vi "ziExample-Module-Sweeper.vi"() -> ()   [LabVIEW 2009]
doc: "Control a Zurich instrument device via the LabOne Labview API. \nRequirements: Zurich Instruments MFLI, HF2 or UHFLI \nThis example shows how to start a sweeper module and retrieve data.\n\n© Zurich Instruments AG, www.zhinst.com"
uses:
  <instrlib>/Zurich Instruments LabOne/Public/Modules/ziTypeModSweeperImpedanceWave.ctl
  <instrlib>/Zurich Instruments LabOne/Public/Modules/ziTypeModSweeperDemodWave.ctl
  <instrlib>/Zurich Instruments LabOne/Public/Modules/ziTypeModSweeperDoubleWave.ctl
  <instrlib>/Zurich Instruments LabOne/Public/Modules/ziModSetValueDouble.vi
  <instrlib>/Zurich Instruments LabOne/Public/Modules/ziModSetValueBinary.vi
  <instrlib>/Zurich Instruments LabOne/Public/Modules/ziModSetValueDoubleArray.vi
  <instrlib>/Zurich Instruments LabOne/Public/Configure/ziSetValueDoubleArray.vi
  <instrlib>/Zurich Instruments LabOne/Public/Modules/ziModGetDoubleData.vi
  <instrlib>/Zurich Instruments LabOne/Public/Modules/ziModGetSweeperData.vi
  <instrlib>/Zurich Instruments LabOne/Zurich Instruments LabOne.lvlib
panel:
  out "SweeperDoubleWaveArray":T1[](array[typedef]) {"bandwidthMode" format="%f"; "flags" format="%f"; "sampleFormat" format="%f"; "sweepMode" format="%f"; "sampleCount" format="%f"; "timestamp" format="%f"}
  out "SweeperDemodWaveArray":T2[](array[typedef]) {"bandwidthMode" format="%f"; "flags" format="%f"; "sampleFormat" format="%f"; "sweepMode" format="%f"; "sampleCount" format="%f"; "timestamp" format="%f"}
  out "SweeperImpedanceWaveArray":T3[](array[typedef]) {"bandwidthMode" format="%f"; "flags" format="%f"; "sampleFormat" format="%f"; "sweepMode" format="%f"; "sampleCount" format="%f"; "timestamp" format="%f"}
  out "Error Out":errorcluster
  in  "Address":string="DEV"
  out "Settings":T4
  out "Selected Device":string
  in  "subscribepath":string="demods/0/sample" caption="Subscribe Path"
  out "Sweeper Phase":cluster{"grid":dbl[], "r_avg":dbl[]}(graph)
  out "Sweeper R":cluster{"grid":dbl[], "r_avg":dbl[]}(graph)
  # "ziExample-SweepModul.vi\nRequirements: HF2LI, UHFLI or MFLI\nsee block diagram for VI description"
  # "Tested Devices:\n- HF2LI\n- UHFLI\n- MFLI"
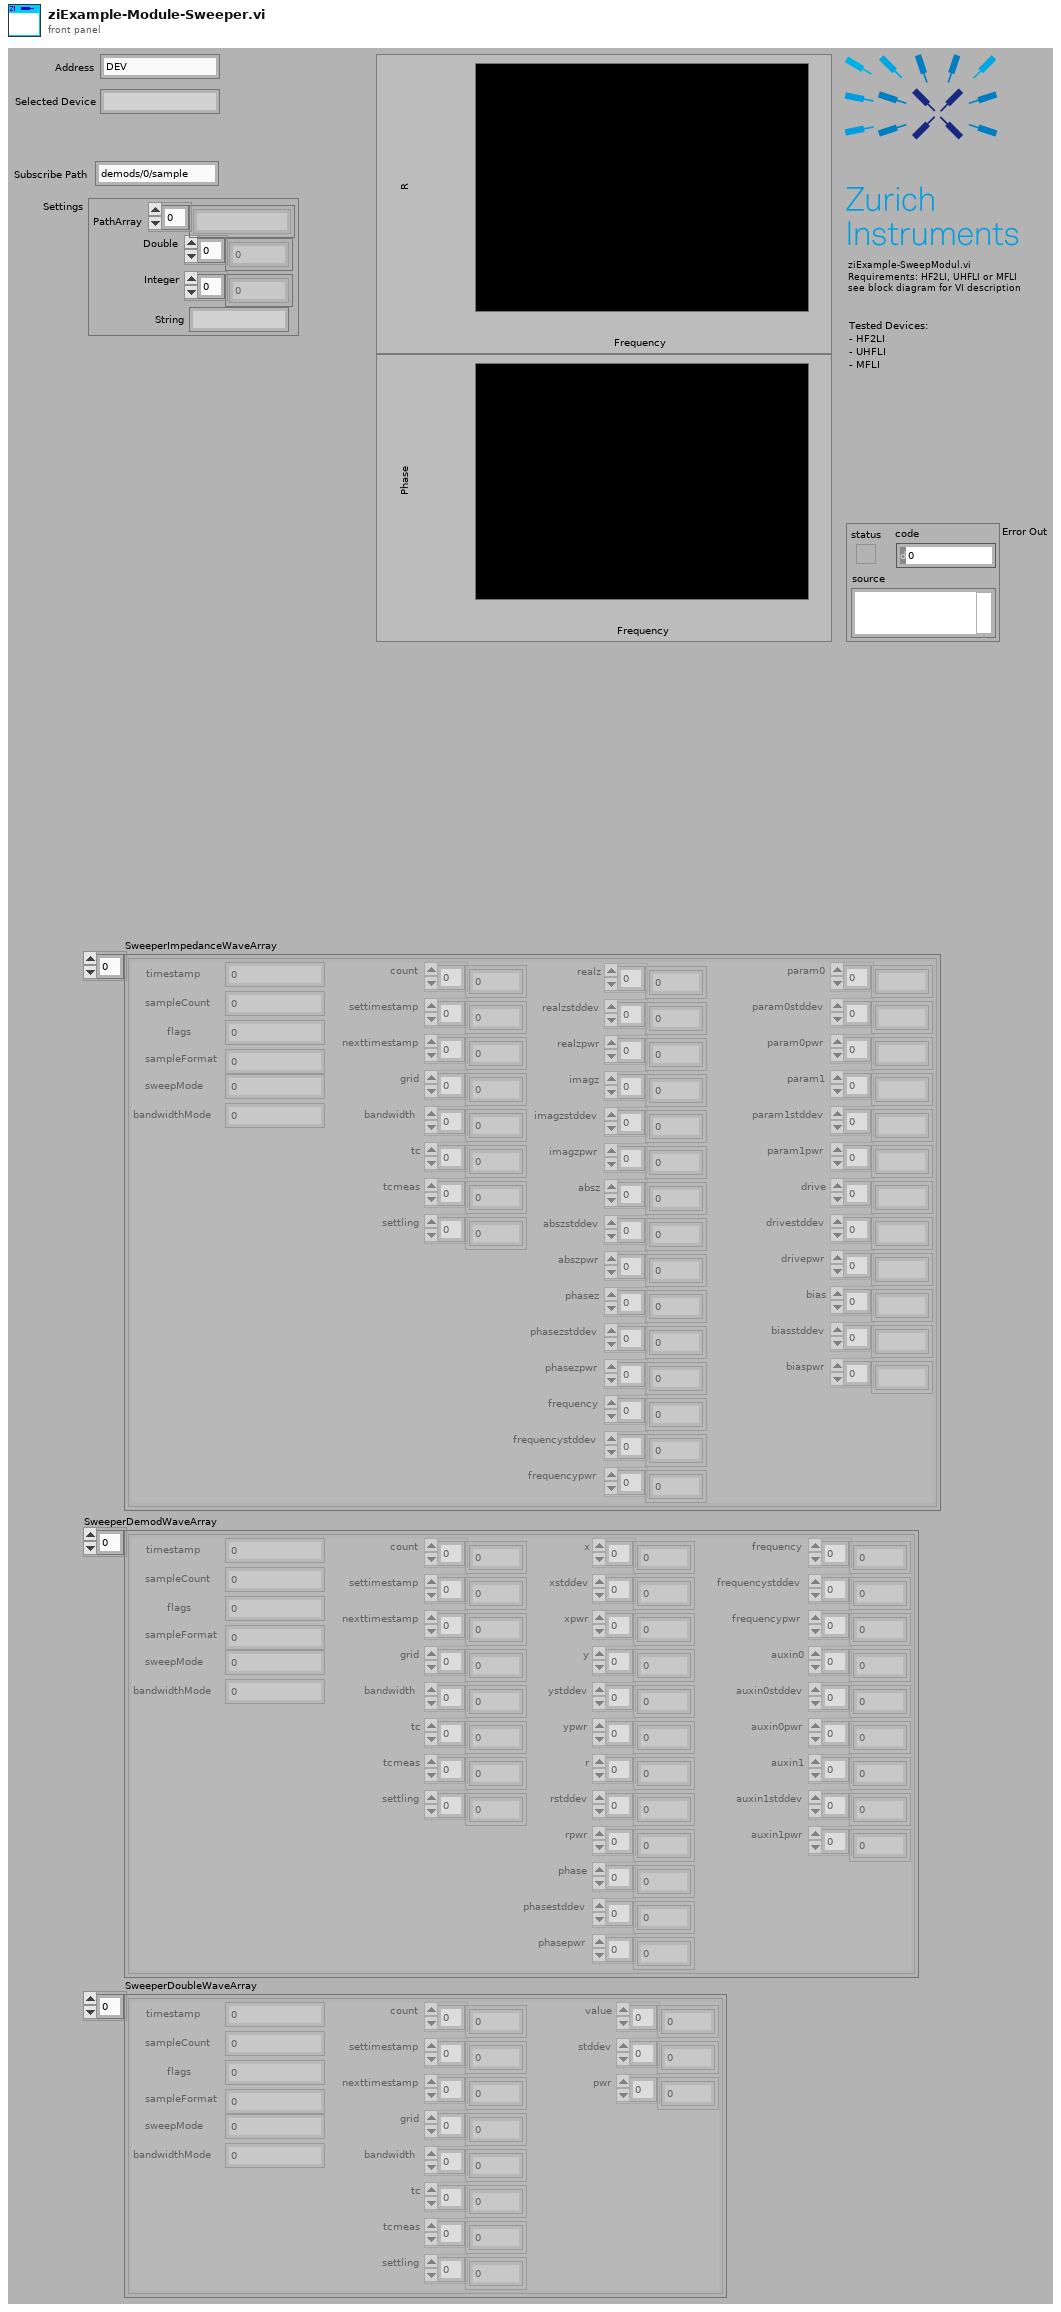
[diagram p1: front panel]
types:
  T1 = typedef "Zurich Instruments LabOne.lvlib/ziTypeModSweeperDoubleWave.ctl" = cluster{"timestamp":u64, "sampleCount":u64, "flags":u8, "sampleFormat":u8, "sweepMode":u8, "bandwidthMode":u8, "count":u64[], "settimestamp":u64[], "nexttimestamp":u64[], "grid":dbl[], "bandwidth":dbl[], "tc":dbl[], "tcmeas":dbl[], "settling":dbl[], "value":dbl[], "stddev":dbl[], "pwr":dbl[]}
  T2 = typedef "Zurich Instruments LabOne.lvlib/ziTypeModSweeperDemodWave.ctl" = cluster{"timestamp":u64, "sampleCount":u64, "flags":u8, "sampleFormat":u8, "sweepMode":u8, "bandwidthMode":u8, "count":u64[], "settimestamp":u64[], "nexttimestamp":u64[], "grid":dbl[], "bandwidth":dbl[], "tc":dbl[], "tcmeas":dbl[], "settling":dbl[], "x":dbl[], "xstddev":dbl[], "xpwr":dbl[], "y":dbl[], "ystddev":dbl[], "ypwr":dbl[], "r":dbl[], "rstddev":dbl[], "rpwr":dbl[], "phase":dbl[], "phasestddev":dbl[], "phasepwr":dbl[], "frequency":dbl[], "frequencystddev":dbl[], "frequencypwr":dbl[], "auxin0":dbl[], "auxin0stddev":dbl[], "auxin0pwr":dbl[], "auxin1":dbl[], "auxin1stddev":dbl[], "auxin1pwr":dbl[]}
  T3 = typedef "Zurich Instruments LabOne.lvlib/ziTypeModSweeperImpedanceWave.ctl" = cluster{"timestamp":u64, "sampleCount":u64, "flags":u8, "sampleFormat":u8, "sweepMode":u8, "bandwidthMode":u8, "count":u64[], "settimestamp":u64[], "nexttimestamp":u64[], "grid":dbl[], "bandwidth":dbl[], "tc":dbl[], "tcmeas":dbl[], "settling":dbl[], "realz":dbl[], "realzstddev":dbl[], "realzpwr":dbl[], "imagz":dbl[], "imagzstddev":dbl[], "imagzpwr":dbl[], "absz":dbl[], "abszstddev":dbl[], "abszpwr":dbl[], "phasez":dbl[], "phasezstddev":dbl[], "phasezpwr":dbl[], "frequency":dbl[], "frequencystddev":dbl[], "frequencypwr":dbl[], "param0":dbl[], "param0stddev":dbl[], "param0pwr":dbl[], "param1":dbl[], "param1stddev":dbl[], "param1pwr":dbl[], "drive":dbl[], "drivestddev":dbl[], "drivepwr":dbl[], "bias":dbl[], "biasstddev":dbl[], "biaspwr":dbl[]}
  T4 = cluster{"String":string, "Integer":dbl[], "Double":dbl[], "PathArray":string[]}
  T5 = typedef "Zurich Instruments LabOne.lvlib/ziTypeHandle.ctl" = cluster{"handleValid":bool, "Conn":u64, "Path Prefix":string, "Handle":u64, "Connected":bool, "Clockbase(s)":dbl}
  T6 = typedef "Zurich Instruments LabOne.lvlib/ziTypeModHandle.ctl" = cluster{"handleValid":bool, "Conn":u64, "ModHandle":u64, "moduleID":string, "Path Prefix":string}
  T7 = cluster{"String":string, "Integer":i64[], "Double":dbl[], "PathArray":string[]}
  T8 = typedef "Zurich Instruments LabOne.lvlib/ziTypeModResults.ctl" = cluster{"PathArray":string[], "ValueType":T9, "NoOfResults":u64, "HeaderType":enum16{"HEADER_TYPE_NONE", "HEADER_TYPE_SWTRIGGER", "HEADER_TYPE_SWEEPER"}, "ziSWTriggerHeader":T10[], "ziSweeperHeader":T11[]}
  T9 = typedef "Zurich Instruments LabOne.lvlib/ziTypePollType.ctl" = enum16{"NONE", "DOUBLE_DATA", "INTEGER_DATA", "DEMOD_SAMPLE", "SCOPE_WAVE_HF2", "AUXIN_SAMPLE", "DIO_SAMPLE", "BYTE_ARRAY", "PWA_WAVE", "9", "10", "11", "12", "13", "14", "15", "TREE_CHANGE_DEPRI", "17", "ERROR", "19", "20", "21", "22", "23", "24", "25", "26", "27", "28", "29", "30", "31", "DOUBLE_DATA_TS", "INTEGER_DATA_TS", "34", "SCOPE_WAVE", "36", "37", "BYTE_ARRAY_TS", "39", "40", "41", "42", "43", "44", "45", "CNT_DATA", "47", "TREE_CHANGE", "49", "50", "51", "52", "53", "54", "55", "56", "57", "58", "59", "60", "61", "62", "63", "SWEEPER_DATA", "SPECTRUM_DATA", "ADVISOR_DATA", "67", "IMP_DATA"}
  T10 = typedef "Zurich Instruments LabOne.lvlib/ziTypeModSWTriggerHeader.ctl" = cluster{"HeaderType":enum8{"HEADER_TYPE_NONE", "HEADER_TYPE_SWTRIGGER", "HEADER_TYPE_SWEEPER"}, "triggerStart":u64, "triggerNumber":u64, "cols":u32, "rows":u32}
  T11 = typedef "Zurich Instruments LabOne.lvlib/ziTypeModSweeperHeader.ctl" = cluster{"HeaderType":enum8{"HEADER_TYPE_NONE", "HEADER_TYPE_SWTRIGGER", "HEADER_TYPE_SWEEPER"}, "sampleFormat":u8}
  T12 = typedef "Zurich Instruments LabOne.lvlib/ziTypeDoubleDataTS.ctl" = cluster{"Timestamp (ticks)":u64[], "Value":dbl[]}
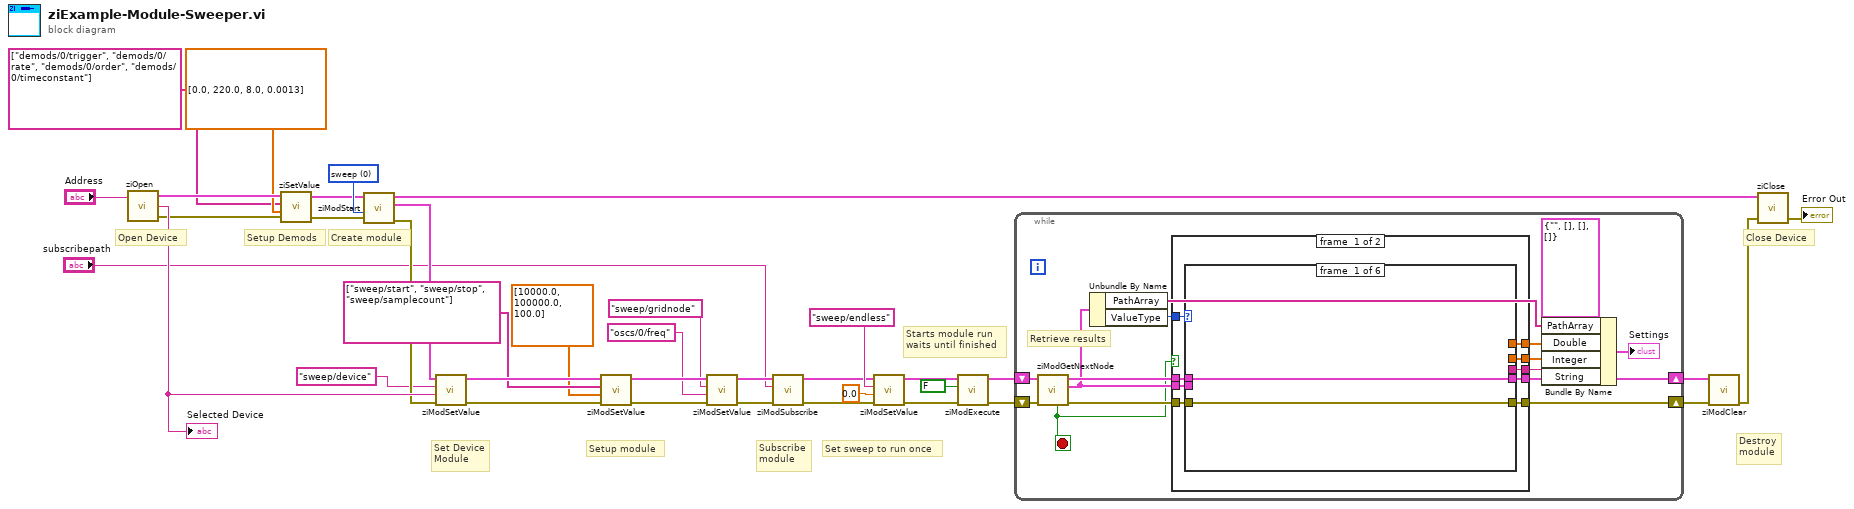
[diagram p0: block diagram]
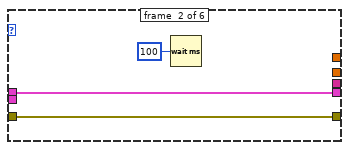
[diagram p2: hidden frame]
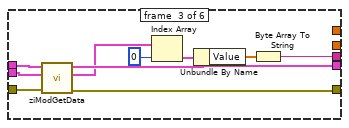
[diagram p3: hidden frame]
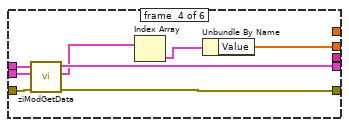
[diagram p4: hidden frame]
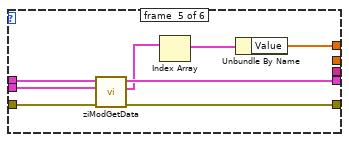
[diagram p5: hidden frame]
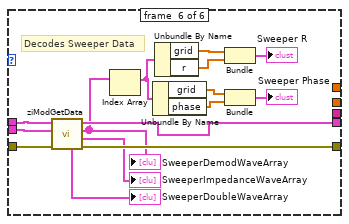
[diagram p6: hidden frame]
diagram:
  w22 = u16 0 items=["sweep", "zoomFFT", "deviceSettings", "record", "pllAdvisor", "pidAdvisor"] ("moduleID")
  # "Setup Demods"
  # "Set Device\nModule"
  # "Destroy\nmodule"
  # "Starts module run\nwaits until finished"
  # "Set sweep to run once"
  # "Subscribe\nmodule"
  # "Setup module"
  # "Create module"
  # "Close Device"
  # "Open Device"
  n1 = call <instrlib>:"ziOpen.vi"("Address"="Address") -> ("Error Out"=w13:errorcluster, "Selected Device"=w36:string, "HandleOut"=w16:T5)  [unwired: 1 in, 2 out]
  "Selected Device" <- w36
  n2 = call-poly <instrlib>:"ziSetValue.vi"("Error In"=w13, "Values"=dbl[] [0.0, 220.0, 8.0, 0.0013], "Paths"=string[] ["demods/0/trigger", "demods/0/rate", "demods/0/order", "demods/0/timeconstant"], "Handle In"=w16) -> ("Error Out"=w14:errorcluster, "Handle Out"=w15:T5)  [unwired: 1 in]
  n3 = call <instrlib>:"ziModStart.vi"("Error In"=w14, "module Id"=w22, "Handle In"=w15) -> ("Error Out"=w20:errorcluster, "ModHandle Out"=w21:T6, "Handle Out"=w35:T5)  [unwired: 6 in]
  n4 = call-poly <instrlib>:"ziModSetValue.vi"("Error In"=w20, "Data"=w36, "Path"="sweep/device", "ModHandle In"=w21) -> ("Error Out"=w19:errorcluster, "ModHandle Out"=w18:T6)  [unwired: 6 in]
  n5 = call-poly <instrlib>:"ziModSetValue.vi"("Error In"=w19, "Values"=dbl[] [10000.0, 100000.0, 100.0], "Paths"=string[] ["sweep/start", "sweep/stop", "sweep/samplecount"], "ModHandle In"=w18) -> ("Error Out"=w32:errorcluster, "ModHandle Out"=w31:T6)  [unwired: 6 in]
  n6 = call-poly <instrlib>:"ziModSetValue.vi"("Error In"=w32, "Data"="oscs/0/freq", "Path"="sweep/gridnode", "ModHandle In"=w31) -> ("Error Out"=w28:errorcluster, "ModHandle Out"=w34:T6)  [unwired: 6 in]
  n7 = call <instrlib>:"ziModSubscribe.vi"("Error In"=w28, "Path"="subscribepath", "ModHandle In"=w34) -> ("Error Out"=w29:errorcluster, "ModHandle Out"=w30:T6)  [unwired: 6 in]
  n8 = call-poly <instrlib>:"ziModSetValue.vi"("Error In"=w29, "Value"=0.0, "Path"="sweep/endless", "ModHandle In"=w30) -> ("Error Out"=w27:errorcluster, "ModHandle Out"=w26:T6)  [unwired: 6 in]
  n9 = call <instrlib>:"ziModExecute.vi"("Error In"=w27, "Modal (F)"=FALSE ("Modal"), "ziModHandle In"=w26) -> ("Error Out"=w23:errorcluster, "ziModHandle Out"=w25:T6)  [unwired: 5 in, 1 out]
  n10 = while {
    shift-right: [w49] -> w2
    shift-left: w25 -> [w51]
    shift-right: [w48] -> w3
    shift-left: w23 -> [w52]
    stop <- w38 stop-if-true
    # "Retrieve results"
    n11 = call <instrlib>:"ziModGetNextNode.vi"("Error In"=w52, "ModHandle In"=w51) -> ("Error Out"=w39:errorcluster, "ModResults"=w47:T8, "ModHandle Out"=w50:T6, "NoData"=w38:bool)  [unwired: 6 in]
    n12 = Unbundle By Name(w47) -> ("PathArray"=w41:string[], "ValueType"=w40:T9)
    n13 = case shown="False" w38 {
      tunnel: w50 -> [w61 w108]
      tunnel: [w60 w108] -> w49
      tunnel: [w59 w109] -> w48
      tunnel: w39 -> [w58 w109]
      tunnel: w47 -> [w57 _]
      tunnel: [w56 _] -> w46
      tunnel: [w55 _] -> w45
      tunnel: [w54 _] -> w44
      tunnel: w40 -> [w53 _]
      frame #0 {
        n14 = case shown="\"SWEEPER_DATA\"" w53 {
          tunnel: w61 -> [w63 w66 w76 w84 w92 w96]
          tunnel: w57 -> [_ _ w75 w83 w91 w107]
          tunnel: w58 -> [w62 w65 w74 w82 w90 w106]
          tunnel: [w62 w65 w73 w81 w88 w105] -> w59
          tunnel: [w63 w66 w72 w80 w89 w104] -> w60
          tunnel: [_ _ w67 _ _ _] -> w56
          tunnel: [_ _ _ w79 _ _] -> w55
          tunnel: [_ _ _ _ w87 _] -> w54
          frame #0 {
          }
          frame #1 {
            n15 = Wait (ms)(milliseconds to wait=u32 100) -> ()  [unwired: 1 out]
          }
          frame #2 {
            n16 = call-poly <instrlib>:"ziModGetData.vi"("Error In"=w74, "ModResults"=w75, "ModHandle In"=w76) -> ("Error Out"=w73:errorcluster, "DoubleSample"=w70:T12[], "ModHandle Out"=w72:T6)  [unwired: 4 in, 2 out]
            n17 = Index Array(array=w70, index=0) -> (element=w69:T12)
            n18 = Unbundle By Name(w69) -> ("Value"=w68:dbl[])
            n19 = Byte Array To String(unsigned byte array=w68) -> (string=w67:string)
          }
          frame #3 {
            n20 = call-poly <instrlib>:"ziModGetData.vi"("Error In"=w82, "ModResults"=w83, "ModHandle In"=w84) -> ("Error Out"=w81:errorcluster, "DoubleSample"=w78:T12[], "ModHandle Out"=w80:T6)  [unwired: 4 in, 2 out]
            n21 = Index Array(array=w78) -> (element=w77:T12)  [unwired: 1 in]
            n22 = Unbundle By Name(w77) -> ("Value"=w79:dbl[])
          }
          frame #4 {
            n23 = call-poly <instrlib>:"ziModGetData.vi"("Error In"=w90, "ModResults"=w91, "ModHandle In"=w92) -> ("Error Out"=w88:errorcluster, "DoubleSample"=w86:T12[], "ModHandle Out"=w89:T6)  [unwired: 4 in, 2 out]
            n24 = Index Array(array=w86) -> (element=w85:T12)  [unwired: 1 in]
            n25 = Unbundle By Name(w85) -> ("Value"=w87:dbl[])
          }
          frame #5 {
            # "Decodes Sweeper Data"
            n26 = call-poly <instrlib>:"ziModGetData.vi"("Error In"=w106, "ModResults"=w107, "ModHandle In"=w96) -> ("Error Out"=w105:errorcluster, "SweeperImpedanceWaveArray"=→"SweeperImpedanceWaveArray":T3[], "SweeperDemodWaveArray"=w95:T2[], "ModHandle Out"=w104:T6, "SweeperDoubleWaveArray"=→"SweeperDoubleWaveArray":T1[])  [unwired: 4 in]
            "SweeperDemodWaveArray" <- w95
            n27 = Index Array(array=w95) -> (element=w97:T2)  [unwired: 1 in]
            n28 = Unbundle By Name(w97) -> ("grid"=w99:dbl[], "phase"=w100:dbl[])
            n29 = Unbundle By Name(w97) -> ("grid"=w102:dbl[], "r"=w103:dbl[])
            n30 = Bundle("grid"=w102, "r"=w103) -> (→"Sweeper R":cluster{"grid":dbl[], "r":dbl[]})  [unwired: 1 in]
            n31 = Bundle("grid"=w99, "phase"=w100) -> (→"Sweeper Phase":cluster{"grid":dbl[], "phase":dbl[]})  [unwired: 1 in]
          }
        }
      }
      frame #1 {
      }
    }
    n32 = Bundle By Name(cluster=T7 {"String"="", "Integer"=[], "Double"=[], "PathArray"=[]} ("Settings 2"), "PathArray"=w41, "Double"=w44, "Integer"=w45, "String"=w46) -> (→"Settings":T7)
  }
  n33 = call <instrlib>:"ziModClear.vi"("Error In"=w3, "ziModHandle In"=w2) -> ("Error Out"=w37:errorcluster)  [unwired: 7 in, 1 out]
  n34 = call <instrlib>:"ziClose.vi"("Error In"=w37, "Handle In"=w35) -> ("Error Out"=→"Error Out":errorcluster)  [unwired: 2 in, 1 out]
